vi "Braitenberg.vi"() -> ()   [LabVIEW 2013]
panel:
  in  "column":i32
  in  "row":i32
  out "Right Sensor":dbl
  out "Left Sensor":dbl
  in  "length 2":i32=3
  in  "length":i32=3
  out "subarray":dbl[][](array[numeric])
  out "Searching":bool
  in  "Stop Search":bool
  in  "Begin Search":bool
  in  "y Start":i32
  in  "x Start":i32
  in  "y Goal":i32
  in  "x Goal":i32
  in  "Stop":bool
  out "Intensity Graph":dbl[][](graph)
  # "X"
  # "Y"
  # "Start"
  # "Goal"
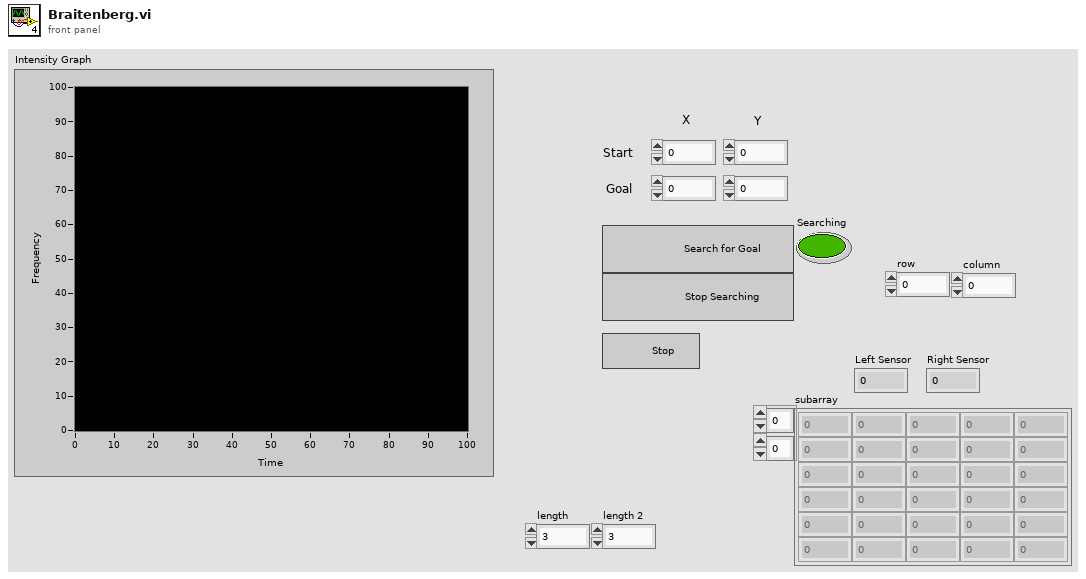
[diagram p1: front panel]
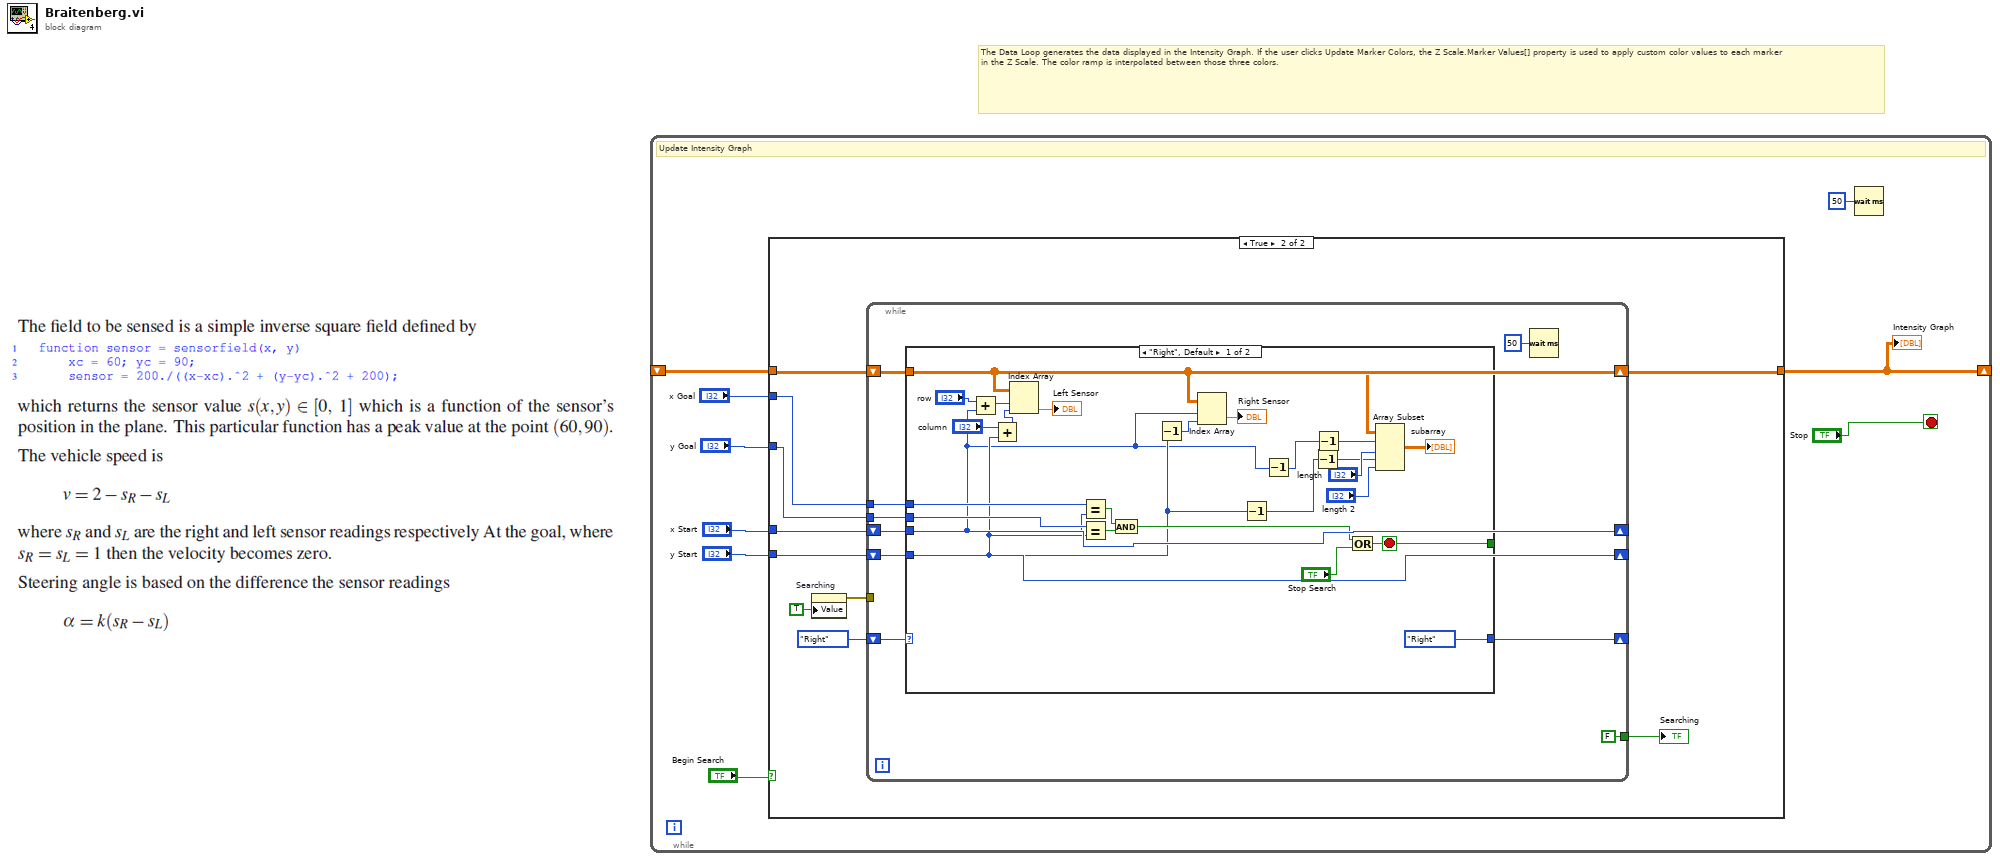
[diagram p0: block diagram]
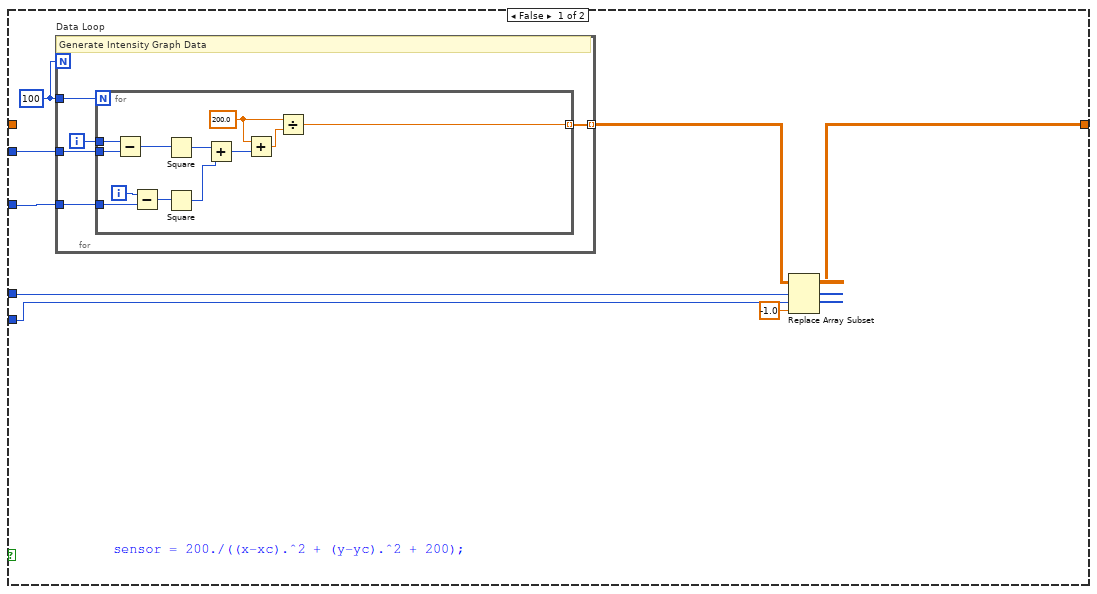
[diagram p2: hidden frame]
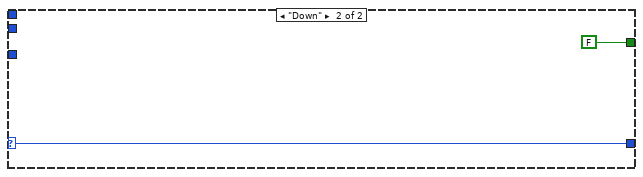
[diagram p3: hidden frame]
diagram:
  # "The Data Loop generates the data displayed in the Intensity Graph. If the user clicks Update Marker Colors, the Z Scale.Marker Values[] property is used to apply custom color values to each marker in the Z Scale. The color ramp is interpolated between those three colors."
  n1 = while {
    shift-right: [w1] -> _
    shift-left: _ -> [w2]
    stop <- "Stop" stop-if-true
    # "Update Intensity Graph"
    n2 = case shown="True" "Begin Search" {
      tunnel: "y Start" -> [w11 w41]
      tunnel: "x Start" -> [w12 w42]
      tunnel: "y Goal" -> [w15 w43]
      tunnel: "x Goal" -> [w16 w44]
      tunnel: w2 -> [_ w40]
      tunnel: [w13 w39] -> w1
      frame False {
        w17 = 100
        n3 = for "Data Loop" {
          N: w17 -> [_]
          tunnel: w17 -> [w22]
          tunnel: [w20] -> w14 mode=indexing
          tunnel: w16 -> [w19]
          tunnel: w15 -> [w18]
          i -> [w21]
          # "Generate Intensity Graph Data"
          n4 = for {
            N: w22 -> [_]
            tunnel: w21 -> [w28]
            tunnel: [w30] -> w20 mode=indexing
            tunnel: w19 -> [w24]
            tunnel: w18 -> [w23]
            i -> [w29]
            w26 = 200.0
            n5 = Subtract(x=w28, y=w24) -> (x-y=w34:i32)
            n6 = Subtract(x=w29, y=w23) -> (x-y=w33:i32)
            n7 = Square(x=w34) -> (x^2=w32:i32)
            n8 = Square(x=w33) -> (x^2=w31:i32)
            n9 = Add(x=w32, y=w31) -> (x+y=w27:i32)
            n10 = Add(x=w26, y=w27) -> (x+y=w25:dbl)
            n11 = Divide(x=w26, y=w25) -> (x/y=w30:dbl)
          }
        }
        n12 = Replace Array Subset(array=w14, new element=-1.0 ("new element/subarray"), index (row)=w12, index (col)=w11) -> (w13:dbl[][])
      }
      frame True {
        n13 = property on="Searching" class="Bool (strict)"("Value"=TRUE ("Searching")) -> (error out=w37:errorcluster)  [unwired: 2 in, 1 out]
        n14 = while {
          tunnel: w44 -> [w54]
          tunnel: w43 -> [w53]
          shift-right: [w49] -> w39
          shift-left: w40 -> [w49]
          shift-right: [w48] -> _
          shift-left: w42 -> [w48]
          shift-right: [w47] -> _
          shift-left: w41 -> [w47]
          tunnel: [FALSE ("Searching")] -> w38
          tunnel: w37 -> [_]
          shift-right: [w46] -> _
          shift-left: enum16{"Right", "Down", "Left", "Up"}."Right" -> [w45]
          stop <- w51 stop-if-true
          n15 = case shown="\"Right\", Default" w45 {
            selector: w45 -> [_ w80]
            tunnel: w54 -> [w79 _]
            tunnel: w53 -> [w76 _]
            tunnel: [w72 FALSE] -> w51
            tunnel: w49 -> [w66 _]
            tunnel: w48 -> [w56 _]
            tunnel: w47 -> [w58 _]
            tunnel: [enum16{"Right", "Down", "Left", "Up"}."Right" w80] -> w46
            frame "Right", Default {
              n16 = Add(x="row", y=w56) -> (x+y=w60:i32)
              n17 = Add(x="column", y=w58) -> (x+y=w59:i32)
              n18 = Index Array(array=w66, index (row)=w60, index (col)=w59) -> (element=→"Left Sensor":dbl)
              n19 = Equal?(x=w79, y=w56) -> (x = y?=w78:bool)
              n20 = Equal?(x=w76, y=w58) -> (x = y?=w77:bool)
              n21 = And(x=w78, y=w77) -> (x .and. y?=w73:bool)
              n22 = Decrement(x=w58) -> (x-1=w64:i32)
              n23 = Index Array(array=w66, index (row)=w56, index (col)=w64) -> (element=→"Right Sensor":dbl)
              n24 = Decrement(x=w58) -> (x-1=w57:i32)
              n25 = Decrement(x=w56) -> (x-1=w55:i32)
              n26 = Decrement(x=w57) -> (x-1=w69:i32)
              n27 = Decrement(x=w55) -> (x-1=w70:i32)
              n28 = Or(x=w73, y="Stop Search") -> (x .or. y?=w72:bool)
              n29 = Array Subset(array=w66, index (row)=w70, length (row)="length", index (col)=w69, length (col)="length 2") -> (→"subarray":dbl[][])
            }
            frame "Down" {
            }
          }
          n30 = Wait (ms)(milliseconds to wait=u32 50) -> ()  [unwired: 1 out]
        }
        "Searching" <- w38
      }
    }
    "Intensity Graph" <- w1
    n31 = Wait (ms)(milliseconds to wait=u32 50) -> ()  [unwired: 1 out]
  }
